vi "Find Hardware.vi"(6 "Remote Timeout (300,000 ms)":u32=300000, 7 "Filter Mode (all values match)":T1=1 items=["all values match"=1, "any value matches"=2, "values do not match"=3, "all properties exist"=4], 8 "error in (no error)":errorcluster, 9 "Experts":string, 10 "Filter in":refnum<k20>, 11 "Session in":refnum<k21>="localhost") -> (0 "error out":errorcluster, 1 "Resources out":refnum<k20>[](array[refnum]), 2 "Filter out":refnum<k20>, 3 "Session out":refnum<k21>)   [LabVIEW 2017, in "nisyscfg.lvlib"]
doc: "Returns a list of hardware in a specified system using the system's session refnum."
uses:
  <vilib>/nisyscfg/nisyscfg.lvlib
  <vilib>/nisyscfg/Filter Mode.ctl
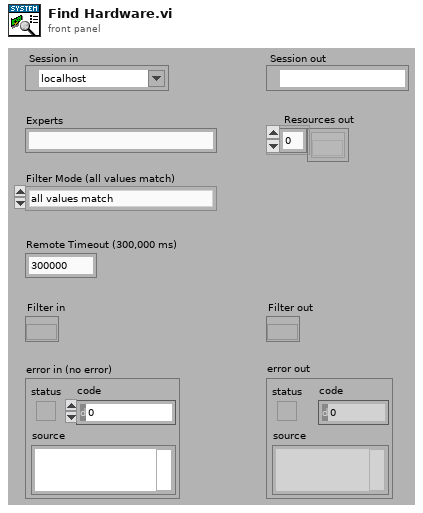
[diagram p1: front panel]
types:
  T1 = typedef "nisyscfg.lvlib/Filter Mode.ctl" = i32
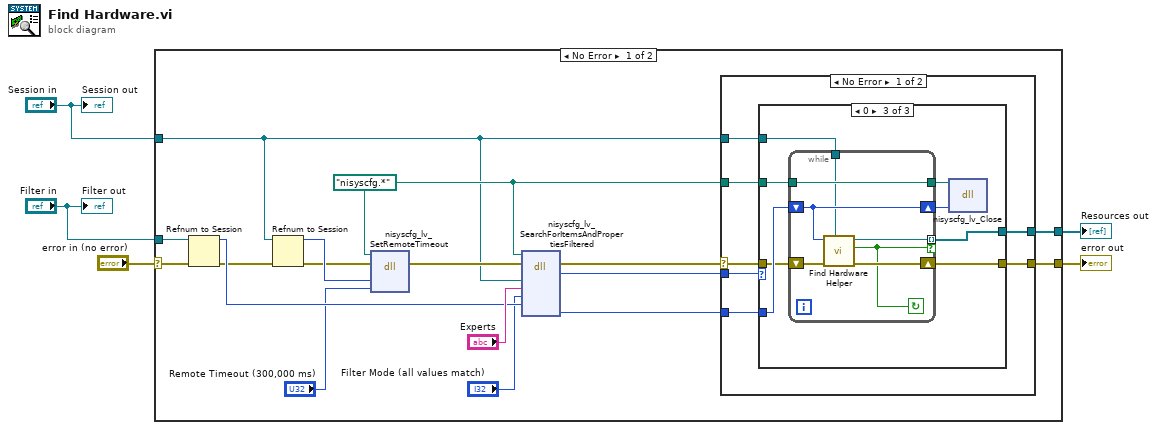
[diagram p0: block diagram]
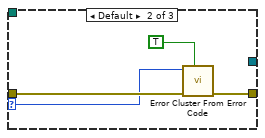
[diagram p3: hidden frame]
diagram:
  n1 = case shown="No Error" "error in (no error)" {
    selector: "error in (no error)" -> [w14 w51]
    tunnel: [w21 w51] -> w5
    tunnel: [w19 _] -> w1
    tunnel: "Session in" -> [w6 _]
    tunnel: "Filter in" -> [w13 _]
    frame No Error {
      w12 = path "nisyscfg.*" ("path in")
      n2 = Refnum to Session(4:w14, 7:w13) -> (0:w8:errorcluster, 3:w18:u64)
      n3 = Refnum to Session(4:w8, 7:w6) -> (0:w7:errorcluster, 3:w9:u64)
      n4 = dll-call lib="nisyscfg.*" fn="nisyscfg_lv_SetRemoteTimeout" label="SetRemoteTimeout"(path in=w12, error in=w7, "item"=w9, "connectTimeout"="Remote Timeout (300,000 ms)") -> (error out=w17:errorcluster)  [unwired: 1 in, 4 out]
      n5 = dll-call lib="nisyscfg.*" fn="nisyscfg_lv_SearchForItemsAndPropertiesFiltered" label="SearchForItemsAndPropertiesFiltered"(path in=w12, error in=w17, "framework"=w6, "experts"="Experts", "filterMode"="Filter Mode (all values match)", "filter"=w18) -> (error out=w11:errorcluster, "status"=w15:i32, "itemsEnum"=w20:u64)  [unwired: 3 in, 4 out]
      n6 = case shown="No Error" w11 {
        selector: w11 -> [w24 w50]
        tunnel: [w29 w50] -> w21
        tunnel: w20 -> [w28 _]
        tunnel: [w27 _] -> w19
        tunnel: w15 -> [w26 _]
        tunnel: w12 -> [w25 _]
        tunnel: w6 -> [w23 _]
        frame No Error {
          n7 = case shown="0" w26 {
            selector: w26 -> [_ w31 _]
            tunnel: [w30 w32 w42] -> w29
            tunnel: w28 -> [_ _ w41]
            tunnel: [_ _ w35] -> w27
            tunnel: w24 -> [w30 w33 w39]
            tunnel: w25 -> [_ _ w38]
            tunnel: w23 -> [_ _ w36]
            frame 1 {
              # "This is S_FALSE which means that\nnothing was found, but it is not an error."
            }
            frame Default {
              n8 = call <vilib>:"Error Cluster From Error Code.vi"("show call chain? (False)"=TRUE, "error in (no error)"=w33, "error code (0)"=w31) -> ("error out"=w32:errorcluster)  [unwired: 6 out]
            }
            frame 0 {
              n9 = while {
                shift-right: [w45] -> w42
                shift-left: w39 -> [w48]
                shift-right: [w47] -> w40
                shift-left: w41 -> [w47]
                tunnel: w38 -> [w49]
                tunnel: [w49] -> w37
                tunnel: w36 -> [w46]
                tunnel: [w44] -> w35 mode=indexing if=w43
                stop <- w43 continue-if-true
                n10 = call <vilib>:"Find Hardware Helper.vi"("Framework"=w46, "error in"=w48, "Enumerator in"=w47) -> ("error out"=w45:errorcluster, "Found Resource"=w43:bool, "Resource out"=w44:refnum<k20>)  [unwired: 6 in]
              }
              n11 = dll-call lib="nisyscfg.*" fn="nisyscfg_lv_Close" label="Close"(path in=w37, "itemsEnum"=w40) -> ()  [unwired: 3 in, 3 out]
            }
          }
        }
        frame Error {
        }
      }
    }
    frame Error {
    }
  }
  "error out" <- w5
  "Resources out" <- w1
  "Session out" <- "Session in"
  "Filter out" <- "Filter in"
